vi "Actor Core.vi"(8 "error in":errorcluster, 11 "Nested in":refnum<class "GUI_Graph.lvclass">) -> (0 "error out":errorcluster, 3 "Actor out":refnum<class "Actor.lvclass">)   [LabVIEW 2020, in "GUI_Graph.lvlib" / "GUI_Graph.lvclass"]
doc: "(<B>Filename</B>: Actor Framework.lvlib:Actor.lvclass:Actor Core.vi)\n\nReceives messages to the actor, reacts to them, and initiates any error handling that may shut the actor down.\n\nDescendant classes may override this VI to append parallel tasks for the actor to complete while it handles messages. Overrides use the Call Parent Method node."
uses:
  GUI_Graph.lvclass
  C:/Program Files/National Instruments/LabVIEW 2020/vi.lib/ActorFramework/Actor/Actor.lvclass
  <vilib>/ActorFramework/Actor/Actor.lvclass
  Measurement/Measurement/Measurement.lvclass
  GUI_Graph.lvclass/GUI_Graph.ctl
  <vilib>/ActorFramework/Actor/Actor.lvclass/Actor.ctl
  <vilib>/ActorFramework/Message Enqueuer/Message Enqueuer.lvclass/Message Enqueuer.ctl
  Measurement/Measurement Messages/Frecuencia Msg/Frecuencia Msg.lvclass/Frecuencia Msg.ctl
  Measurement/Measurement Messages/Amplitud Msg/Amplitud Msg.lvclass/Amplitud Msg.ctl
  Measurement/Measurement Messages/Signal type Msg/Signal type Msg.lvclass/Signal type Msg.ctl
  Measurement/Measurement Messages/START STOP Msg/START STOP Msg.lvclass/START STOP Msg.ctl
  GUI_Graph Messages/Start Stop Msg/Start Stop Msg.lvclass/Start Stop Msg.ctl
  GUI_Graph Messages/Log enable Msg/Log enable Msg.lvclass/Log enable Msg.ctl
  GUI_Graph Messages/File Path Msg/File Path Msg.lvclass/File Path Msg.ctl
  GUI_Graph Messages/file format Msg/file format Msg.lvclass/file format Msg.ctl
  <vilib>/ActorFramework/Message Enqueuer/Init from Existing Queue.vi
  <vilib>/ActorFramework/Message Enqueuer/Enqueue.vi
  <vilib>/ActorFramework/Stop Msg/Stop Msg.lvclass
  C:/Program Files/National Instruments/LabVIEW 2020/vi.lib/ActorFramework/Message/Message.lvclass
  Measurement/Measurement Messages/Frecuencia Msg/Frecuencia Msg.lvclass
  Measurement/Measurement Messages/Amplitud Msg/Amplitud Msg.lvclass
  Measurement/Measurement Messages/Signal type Msg/Signal type Msg.lvclass
  Measurement/Measurement Messages/START STOP Msg/START STOP Msg.lvclass
  GUI_Graph Messages/Start Stop Msg/Start Stop Msg.lvclass
  GUI_Graph Messages/Log enable Msg/Log enable Msg.lvclass
  GUI_Graph Messages/File Path Msg/File Path Msg.lvclass
  GUI_Graph Messages/file format Msg/file format Msg.lvclass
  <vilib>/ActorFramework/Message Priority Queue/Priority Enqueue.vi
  <vilib>/ActorFramework/Message Enqueuer/Message Enqueuer.lvclass
panel:
  out "Waveform Chart":waveform(dbl)(graph)
  in  "Amplitud":dbl(slide) scale=0.0..10.0
  in  "Frecuencia":dbl(slide) scale=0.0..10.0
  in  "Signal":u16(ring) items=["Senoidal", "Triangular", "Cuadrado"]
  in  "Tipo de archivo":enum16{"TXT", "BIN"}(ring) caption="Enum 3"
  in  "File Path":path
  in  "Save":bool
  in  "Stop Button":bool
  in  "Play Button":bool
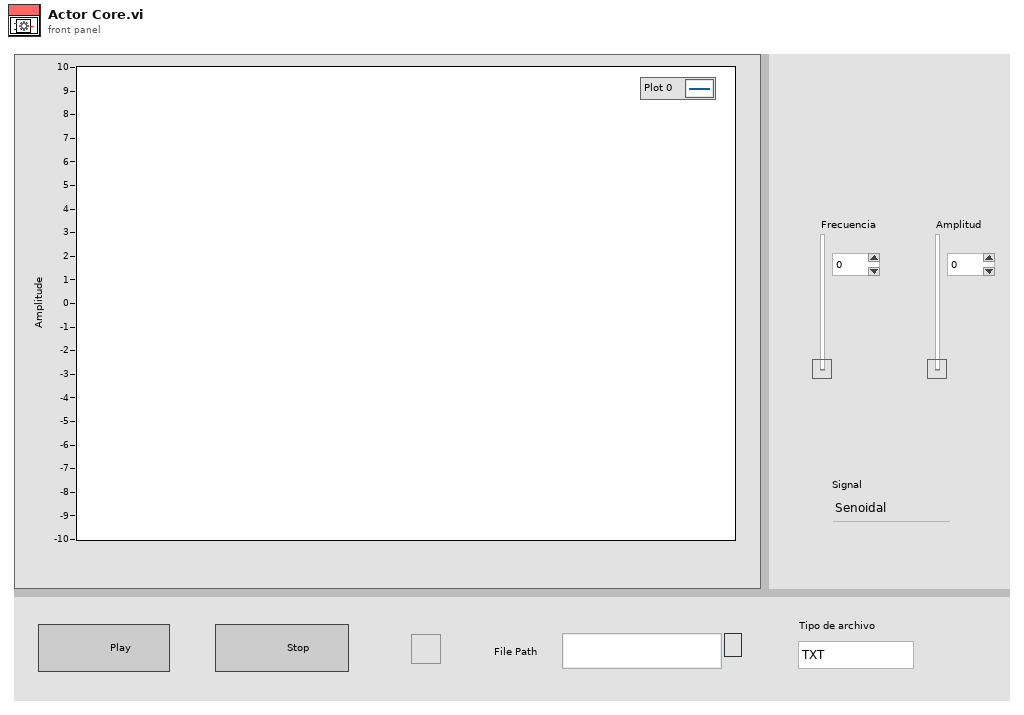
[diagram p1: front panel]
types:
  T1 = cluster{"Stop":refnum<user-event>, "Graph Data":refnum<user-event>}
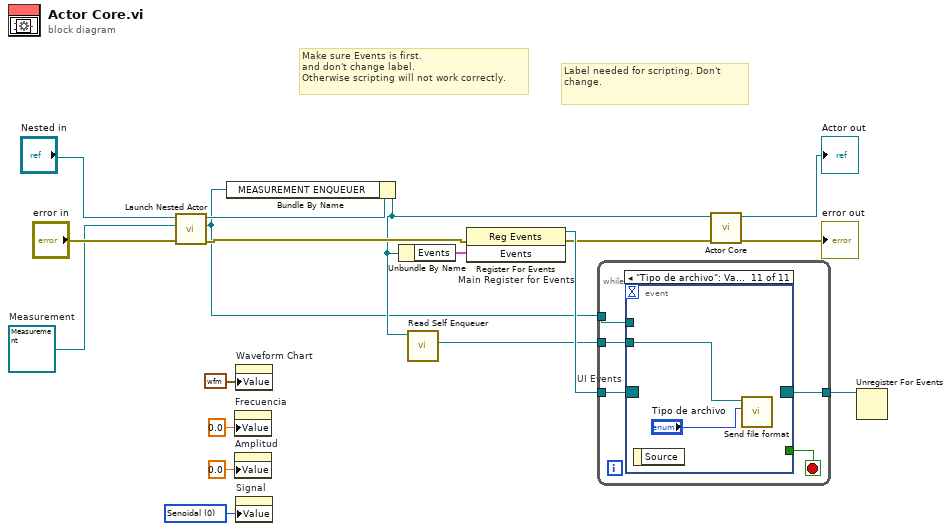
[diagram p0: block diagram]
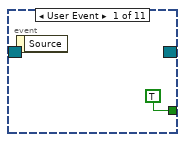
[diagram p2: hidden frame]
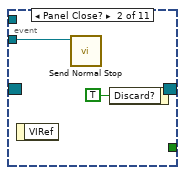
[diagram p3: hidden frame]
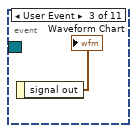
[diagram p4: hidden frame]
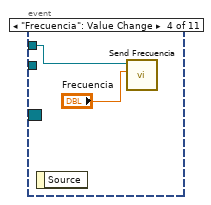
[diagram p5: hidden frame]
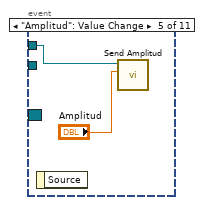
[diagram p6: hidden frame]
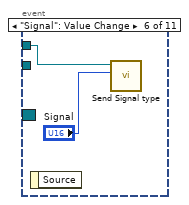
[diagram p7: hidden frame]
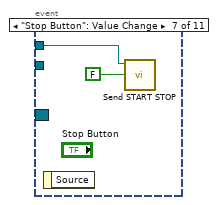
[diagram p8: hidden frame]
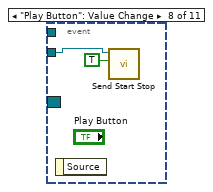
[diagram p9: hidden frame]
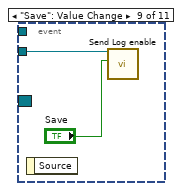
[diagram p10: hidden frame]
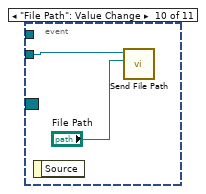
[diagram p11: hidden frame]
diagram:
  w1 = u16 0 items=["Senoidal", "Triangular", "Cuadrado"] ("Signal")
  w7 = refnum<class "Measurement.lvclass"> refnum  # Measurement
  # "Label needed for scripting. Don't change."
  # "Make sure Events is first.\nand don't change label.\nOtherwise scripting will not work correctly."
  n1 = call <vilib>:"Launch Nested Actor.vi"("error in (no error)"="error in", "Nested Actor"=w7, "Caller Actor in"="Nested in") -> ("error out"=w10:errorcluster, "Nested Actor's Enqueuer"=w5:refnum<class "Message Enqueuer.lvclass">, "Caller Actor out"=w8:refnum<class "GUI_Graph.lvclass">)  [unwired: 6 in]
  n2 = Bundle By Name(cluster=w8, "MEASUREMENT ENQUEUER"=w5) -> (w6:refnum<class "GUI_Graph.lvclass">)
  n3 = property on="Frecuencia" class="Slide (strict)"("Value"=0.0 ("Frecuencia")) -> ()  [unwired: 2 in, 2 out]
  n4 = property on="Amplitud" class="Slide (strict)"("Value"=0.0 ("Amplitud")) -> ()  [unwired: 2 in, 2 out]
  n5 = property on="Waveform Chart" class="WFChart (strict)"("Value"=waveform(dbl) {"t0"=timestamp(0 s since 1904-01-01), "dt"=1.0, "Y"=[]} ("Waveform Chart")) -> ()  [unwired: 2 in, 2 out]
  n6 = property on="Signal" class="Ring (strict)"("Value"=w1) -> ()  [unwired: 2 in, 2 out]
  n7 = Unbundle By Name(w6) -> ("Events"=w15:T1)
  n8 = call <vilib>:"Read Self Enqueuer.vi"("Actor"=w6) -> ("Self Enqueuer"=w13:refnum<class "Message Enqueuer.lvclass">)  [unwired: 10 in]
  n9 = register-events "Main Register for Events"(error in=w10, w15) -> (reference out=w16:refnum<event-registration>, error out=w12:errorcluster)  [unwired: 1 in]
  n10 = while {
    tunnel: w16 -> [w23]
    tunnel: [w21] -> w14
    tunnel: w13 -> [w20]
    tunnel: w5 -> [w19]
    stop <- w22 stop-if-true
    n11 = event "UI Events" shown="[10] \"Tipo de archivo\": Value Change" {
      selector: w23 -> [_ _ _ _ _ _ _ _ _ _ _]
      dyn-events: [_ _ _ _ _ _ _ _ _ _ _] -> w21
      timeout: _ -> [_ _ _ _ _ _ _ _ _ _ _]
      tunnel: [TRUE _ _ _ _ _ _ _ _ _ _] -> w22
      tunnel: w20 -> [_ w25 _ _ _ _ _ w36 w39 w41 w43]
      tunnel: w19 -> [_ _ _ w28 w30 w32 w34 _ _ _ _]
      event User Event {
        n12 = event-data() -> ()  [unwired: 1 in, 1 out]
      }
      event Panel Close? {
        n13 = event-data() -> ()  [unwired: 1 in, 1 out]
        n14 = call <vilib>:"Send Normal Stop.vi"("Message Enqueuer"=w25) -> ()  [unwired: 10 in, 1 out]
        n15 = event-data("Discard?"=TRUE) -> ()  [unwired: 1 in, 1 out]
      }
      event User Event {
        n16 = event-data() -> ("signal out"=→"Waveform Chart":waveform(dbl))  [unwired: 1 in]
      }
      event "Frecuencia": Value Change {
        n17 = event-data() -> ()  [unwired: 1 in, 1 out]
        n18 = call "Send Frecuencia.vi"("Frecuencia"="Frecuencia", "Message Enqueuer"=w28) -> ()  [unwired: 8 in, 2 out]
      }
      event "Amplitud": Value Change {
        n19 = event-data() -> ()  [unwired: 1 in, 1 out]
        n20 = call "Send Amplitud.vi"("Amplitud"="Amplitud", "Message Enqueuer"=w30) -> ()  [unwired: 8 in, 2 out]
      }
      event "Signal": Value Change {
        n21 = event-data() -> ()  [unwired: 1 in, 1 out]
        n22 = call "Send Signal type.vi"("signal"="Signal", "Message Enqueuer"=w32) -> ()  [unwired: 8 in, 2 out]
      }
      event "Stop Button": Value Change {
        n23 = event-data() -> ()  [unwired: 1 in, 1 out]
        n24 = call "Send START STOP.vi"("Start/stop"=FALSE, "Message Enqueuer"=w34) -> ()  [unwired: 8 in, 2 out]
      }
      event "Play Button": Value Change {
        n25 = event-data() -> ()  [unwired: 1 in, 1 out]
        n26 = call "Send Start Stop.vi"("Start/stop"=TRUE, "Message Enqueuer"=w36) -> ()  [unwired: 8 in, 2 out]
      }
      event "Save": Value Change {
        n27 = event-data() -> ()  [unwired: 1 in, 1 out]
        n28 = call "Send Log enable.vi"("Log"="Save", "Message Enqueuer"=w39) -> ()  [unwired: 8 in, 2 out]
      }
      event "File Path": Value Change {
        n29 = event-data() -> ()  [unwired: 1 in, 1 out]
        n30 = call "Send File Path.vi"("Path"="File Path", "Message Enqueuer"=w41) -> ()  [unwired: 8 in, 2 out]
      }
      event "Tipo de archivo": Value Change {
        n31 = event-data() -> ()  [unwired: 1 in, 1 out]
        n32 = call "Send file format.vi"("Tipo de archivo"="Tipo de archivo", "Message Enqueuer"=w43) -> ()  [unwired: 8 in, 2 out]
      }
    }
  }
  n33 = call-parent "Actor Core.vi"("error in"=w12, "Actor in"=w6) -> ("error out"=→"error out":errorcluster, "Actor out"=→"Actor out":refnum<class "Actor.lvclass">)  [unwired: 8 in]
  n34 = Unregister For Events(event registration refnum=w14) -> ()  [unwired: 1 in, 1 out]
